vi "FlowPlotResults.vi"(8 "error in (no error)":errorcluster, 9 "Text":dbl, 10 "Cluster":T1, 11 "Graph":refnum<vi>) -> (0 "error out":errorcluster, 3 "reference out":refnum<vi>)   [LabVIEW 2013, in "main.lvlib"]
uses:
  main.lvlib
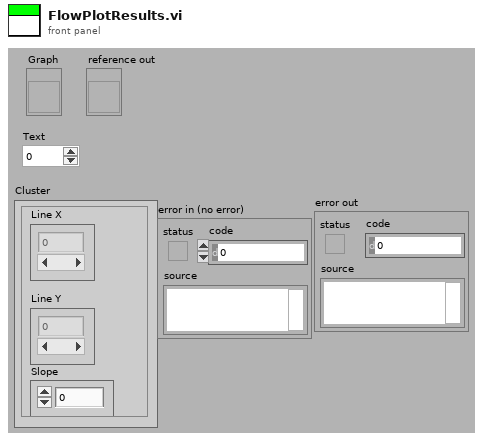
[diagram p1: front panel]
types:
  T1 = cluster{"Line X":dbl[], "Line Y":dbl[], "Slope":dbl}
  T2 = cluster{"Font Name:":string, "Size":i16, "Strikeout?":bool, "Italic?":bool, "Underline?":bool, "Outline?":bool, "Shadow?":bool, "Bold?":bool}
  T3 = enum16{"User-specified Font", "Application Font", "System Font", "Dialog Font"}
  T4 = cluster{"horizontal":enum16{"left", "center", "right"}, "vertical":enum16{"top", "center", "bottom"}}
  T5 = typedef "LVBoundsTypeDef.ctl" = cluster{"Width":u32, "Height":u32}
  T6 = cluster{"Array out":dbl[], "Best Linear Fit":dbl[]}[]
  T7 = typedef "LVRectTypeDef.ctl" = cluster{"Left":i16, "Top":i16, "Right":i16, "Bottom":i16}
  T8 = cluster{"Array out":dbl[], "Best Linear Fit":dbl[]}
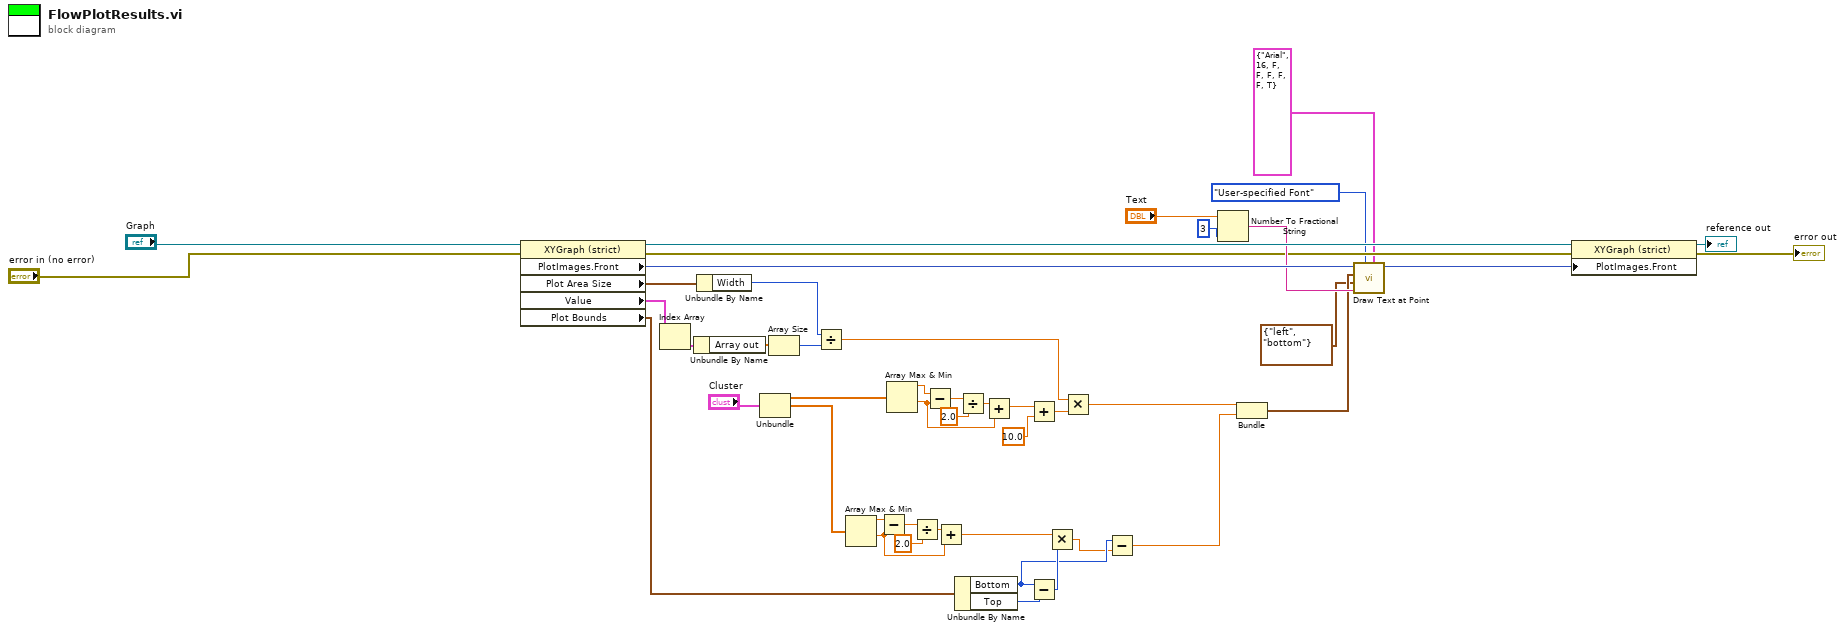
[diagram p0: block diagram]
diagram:
  n1 = property class="XYGraph (strict)"(reference="Graph", error in="error in (no error)") -> (reference out=w45:refnum<vi>, error out=w43:errorcluster, "PlotImages.Front"=w46:picture, "Plot Area Size"=w27:T5, "Value"=w26:T6, "Plot Bounds"=w1:T7)
  n2 = Index Array(array=w26) -> (element=w25:T8)  [unwired: 1 in]
  n3 = Unbundle By Name(w25) -> ("Array out"=w23:dbl[])
  n4 = Unbundle By Name(w27) -> ("Width"=w3:u32)
  n5 = Unbundle("Cluster") -> ("Line X"=w35:dbl[], "Line Y"=w36:dbl[])  [unwired: 1 out]
  n6 = Array Size(array=w23) -> (size(s)=w22:i32)
  n7 = Divide(x=w3, y=w22) -> (x/y=w24:dbl)
  n8 = Array Max & Min(array=w36) -> (max value=w40:dbl, min value=w28:dbl)  [unwired: 2 out]
  n9 = Subtract(x=w40, y=w28) -> (x-y=w39:dbl)
  n10 = Array Max & Min(array=w35) -> (max value=w32:dbl, min value=w30:dbl)  [unwired: 2 out]
  n11 = Divide(x=w39, y=2.0) -> (x/y=w37:dbl)
  n12 = Subtract(x=w32, y=w30) -> (x-y=w34:dbl)
  n13 = Add(x=w37, y=w28) -> (x+y=w4:dbl)
  n14 = Unbundle By Name(w1) -> ("Bottom"=w8:i16, "Top"=w20:i16)
  n15 = Divide(x=w34, y=2.0) -> (x/y=w31:dbl)
  n16 = Add(x=w31, y=w30) -> (x+y=w17:dbl)
  n17 = Add(x=w17, y=10.0) -> (x+y=w18:dbl)
  n18 = Subtract(x=w8, y=w20) -> (x-y=w21:i16)
  n19 = Multiply(x=w4, y=w21) -> (x*y=w7:dbl)
  n20 = Multiply(x=w24, y=w18) -> (x*y=w2:dbl)
  n21 = Subtract(x=w8, y=w7) -> (x-y=w19:dbl)
  n22 = Number To Fractional String(number="Text", precision (6)=i16 3 ("width (-)")) -> (F-format string=w44:string)  [unwired: 2 in]
  n23 = Bundle(w2, w19) -> (w14:cluster{dbl, dbl})  [unwired: 1 in]
  n24 = call <vilib>:"Draw Text at Point.vi"("[user-specified font]"=T2 {"Font Name:"="Arial", "Size"=16, "Strikeout?"=FALSE, "Italic?"=FALSE, "Underline?"=FALSE, "Outline?"=FALSE, "Shadow?"=FALSE, "Bold?"=TRUE}, "desired font(Application)"=T3."User-specified Font", "text"=w44, "alignment(left, top)"=T4 {"horizontal"=enum."left", "vertical"=enum."bottom"}, "origin"=w14, "picture"=w46) -> ("new picture"=w10:picture)  [unwired: 4 in, 1 out]
  n25 = property class="XYGraph (strict)"(reference=w45, error in=w43, "PlotImages.Front"=w10) -> (reference out=→"reference out":refnum<vi>, error out=→"error out":errorcluster)
